vi "ReadIO.vi"(0 "ArrayPairs In":T5={"iStatus"={"Index"=0, "Value"=0.0}, "TIME"={"Index"=1, "Value"=0.0}, "DT"={"Index"=2, "Value"=0.0}, "Blade1PitchPos_rad"={"Index"=3, "Value"=0.0}, "VS_MECHGENPWR"={"Index"=13, "Value"=0.0}, "VS_GENPWR"={"Index"=14, "Value"=0.0}, "GEN_SPEED"={"Index"=19, "Value"=0.0}, "ROTOR_SPEED"={"Index"=20, "Value"=0.0}, "GENTQMEAS"={"Index"=22, "Value"=0.0}, "Y_M"={"Index"=23, "Value"=0.0}, "HORWINDV"={"Index"=26, "Value"=0.0}, "ROOTMOOP1"={"Index"=29, "Value"=0.0}, "ROOTMOOP2"={"Index"=30, "Value"=0.0}, "Blade2PitchPos_rad"={"Index"=32, "Value"=0.0}, "Blade3PitchPos_rad"={"Index"=33, "Value"=0.0}, "ROOTMOOP3"={"Index"=31, "Value"=0.0}, "AVCMSG_SIZE"={"Index"=48, "Value"=0.0}, "INFILE_SIZE "={"Index"=49, "Value"=0.0}, "OUTFILE_SIZE "={"Index"=50, "Value"=0.0}, "FA_ACC"={"Index"=52, "Value"=0.0}, "NUM_BLADES"={"Index"=60, "Value"=0.0}, "BladePitchSetpoint_rad"={"Index"=44, "Value"=0.0}, "TorqueSetpoint_Nm"={"Index"=46, "Value"=0.0}, "OUT_AEROTQ"={"Index"=89, "Value"=0.0}, "Out.RotSpeed "={"Index"=92, "Value"=0.0}, "Out.DEBUG"={"Index"=93, "Value"=0.0}}, 1 "PitchAxis1State":T2, 2 "PitchAxis2State":T2, 3 "PitchAxis3State":T2, 5 "IO Signals In":T3, 9 "ROSCO Params In":T4, 11 "error in":errorcluster, 12 "zeroRotorPos":bool) -> (4 "ArrayPairs Out":T5={"iStatus"={"Index"=0, "Value"=0.0}, "TIME"={"Index"=1, "Value"=0.0}, "DT"={"Index"=2, "Value"=0.0}, "Blade1PitchPos_rad"={"Index"=3, "Value"=0.0}, "VS_MECHGENPWR"={"Index"=13, "Value"=0.0}, "VS_GENPWR"={"Index"=14, "Value"=0.0}, "GEN_SPEED"={"Index"=19, "Value"=0.0}, "ROTOR_SPEED"={"Index"=20, "Value"=0.0}, "GENTQMEAS"={"Index"=22, "Value"=0.0}, "Y_M"={"Index"=23, "Value"=0.0}, "HORWINDV"={"Index"=26, "Value"=0.0}, "ROOTMOOP1"={"Index"=29, "Value"=0.0}, "ROOTMOOP2"={"Index"=30, "Value"=0.0}, "Blade2PitchPos_rad"={"Index"=32, "Value"=0.0}, "Blade3PitchPos_rad"={"Index"=33, "Value"=0.0}, "ROOTMOOP3"={"Index"=31, "Value"=0.0}, "AVCMSG_SIZE"={"Index"=48, "Value"=0.0}, "INFILE_SIZE "={"Index"=49, "Value"=0.0}, "OUTFILE_SIZE "={"Index"=50, "Value"=0.0}, "FA_ACC"={"Index"=52, "Value"=0.0}, "NUM_BLADES"={"Index"=60, "Value"=0.0}, "BladePitchSetpoint_rad"={"Index"=44, "Value"=0.0}, "TorqueSetpoint_Nm"={"Index"=46, "Value"=0.0}, "OUT_AEROTQ"={"Index"=89, "Value"=0.0}, "Out.RotSpeed "={"Index"=92, "Value"=0.0}, "Out.DEBUG"={"Index"=93, "Value"=0.0}}, 6 "IO Signals Out":T3, 10 "ROSCO Params Out":T4, 14 "Torque RAW (V)":dbl, 15 "error out":errorcluster)   [LabVIEW 2018]
uses:
  Clusters/ArrayPairs.ctl
  Clusters/SwapArrayCluster.ctl
  Clusters/RoscoParams.ctl
  Clusters/IOSignals.ctl
  Clusters/ElmoState.ctl
  Clusters/AnemometerData.ctl
  Clusters/SimulationConstants.ctl
panel:
  in  "Anemometer Data":T1
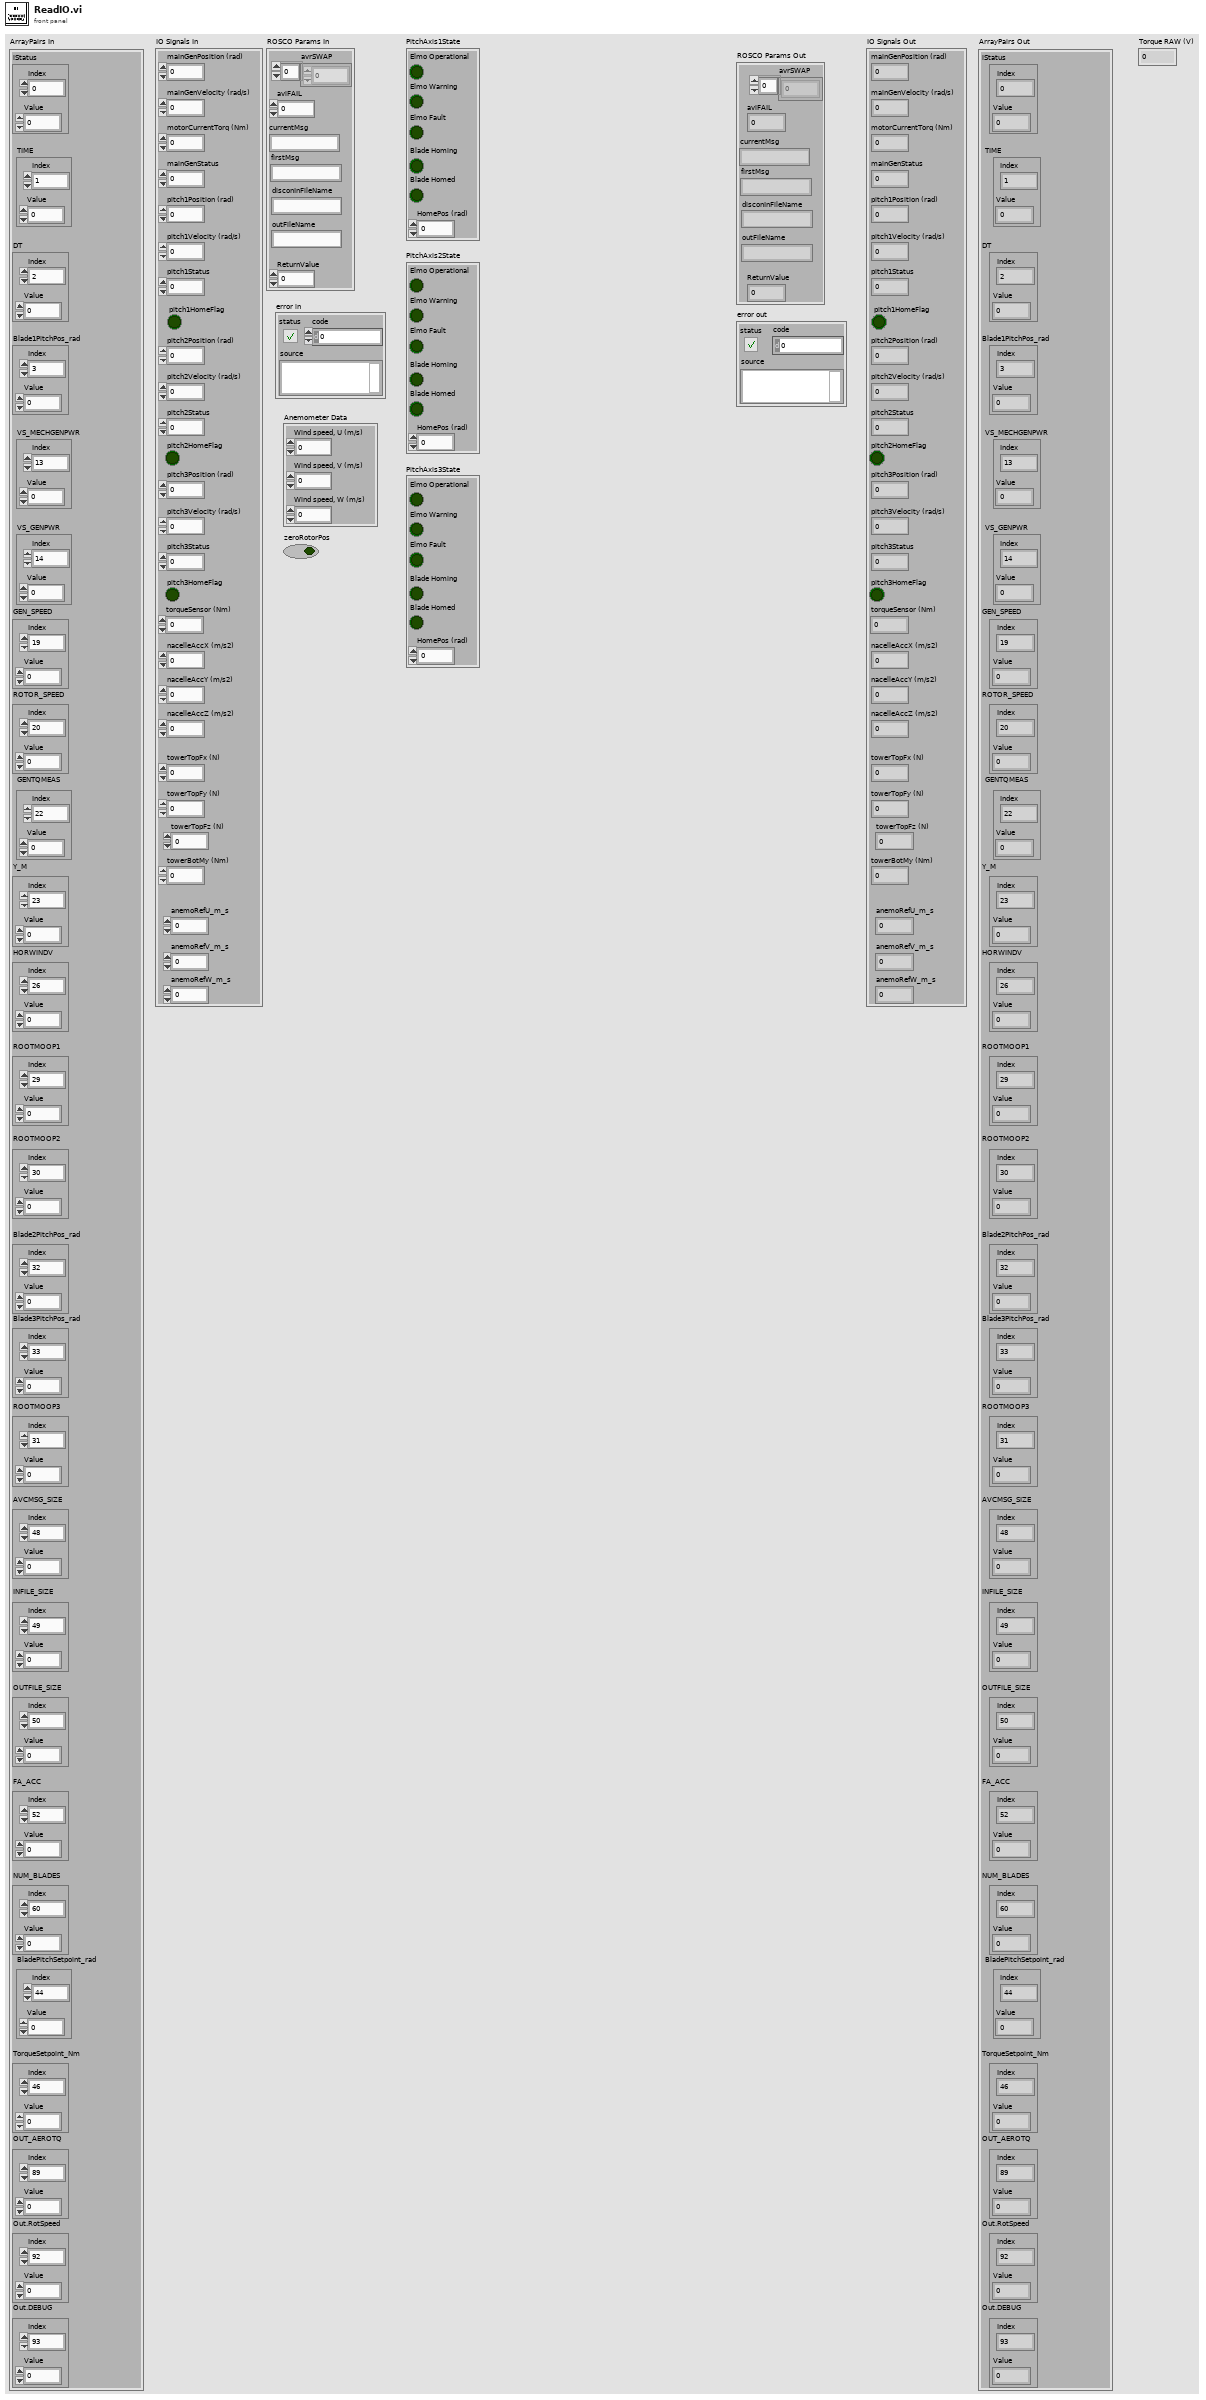
[diagram p1: front panel]
types:
  T1 = typedef "AnemometerData.ctl" = cluster{"Wind speed, U (m/s)":dbl, "Wind speed, V (m/s)":dbl, "Wind speed, W (m/s)":dbl}
  T2 = typedef "ElmoState.ctl" = cluster{"Elmo Operational":bool, "Elmo Warning":bool, "Elmo Fault":bool, "Blade Homed":bool, "Blade Homing":bool, "HomePos (rad)":dbl}
  T3 = typedef "IOSignals.ctl" = cluster{"mainGenPosition (rad)":dbl, "motorCurrentTorq (Nm)":dbl, "mainGenVelocity (rad/s)":dbl, "mainGenStatus":u16, "pitch1Position (rad)":dbl, "pitch1Velocity (rad/s)":dbl, "pitch1Status":u16, "pitch2Position (rad)":dbl, "pitch2Velocity (rad/s)":dbl, "pitch2Status":u16, "pitch3Position (rad)":dbl, "pitch3Velocity (rad/s)":dbl, "pitch3Status":u16, "torqueSensor (Nm)":dbl, "nacelleAccX (m/s2)":dbl, "nacelleAccY (m/s2)":dbl, "nacelleAccZ (m/s2)":dbl, "pitch1HomeFlag":bool, "pitch2HomeFlag":bool, "pitch3HomeFlag":bool, "towerTopFx (N)":dbl, "towerTopFy (N)":dbl, "towerTopFz (N)":dbl, "towerBotMy (Nm)":dbl, "anemoRefU_m_s":dbl, "anemoRefV_m_s":dbl, "anemoRefW_m_s":dbl}
  T4 = typedef "RoscoParams.ctl" = cluster{"avrSWAP":dbl[], "aviFAIL":i32, "currentMsg":string, "ReturnValue":i32, "disconInFileName":string, "outFileName":string, "firstMsg":string}
  T5 = typedef "ArrayPairs.ctl" = cluster{"iStatus":T6, "TIME":T6, "DT":T6, "Blade1PitchPos_rad":T6, "VS_MECHGENPWR":T6, "VS_GENPWR":T6, "GEN_SPEED":T6, "ROTOR_SPEED":T6, "GENTQMEAS":T6, "Y_M":T6, "HORWINDV":T6, "ROOTMOOP1":T6, "ROOTMOOP2":T6, "Blade2PitchPos_rad":T6, "Blade3PitchPos_rad":T6, "ROOTMOOP3":T6, "AVCMSG_SIZE":T6, "INFILE_SIZE ":T6, "OUTFILE_SIZE ":T6, "FA_ACC":T6, "NUM_BLADES":T6, "BladePitchSetpoint_rad":T6, "TorqueSetpoint_Nm":T6, "OUT_AEROTQ":T6, "Out.RotSpeed ":T6, "Out.DEBUG":T6}
  T6 = typedef "SwapArrayCluster.ctl" = cluster{"Index":i32, "Value":dbl}
  T7 = typedef "SimulationConstants.ctl" = cluster{"nGear":dbl, "rotorRadius":sgl, "numBlades":i32, "scaleFactor":dbl, "roscoInitMinSpeed_rad_s":dbl, "roscoInitMinTorqueFS_Nm":dbl, "beckhoff16bit":dbl, "beckhoff24BitExt":i32, "BX824Bit":i32, "rotorTorqueScale_Nm_V":dbl, "rotorTorqueOfst_Nm":dbl, "rangeEL3104V":dbl, "nacelleAccELM3604V":dbl, "nacelleAccScaleX_m_s2_V":dbl, "nacelleAccOfstX_m_s2":dbl, "nacelleAccScaleY_m_s2_V":dbl, "nacelleAccOfstY_m_s2":dbl, "nacelleAccScaleZ_m_s2_V":dbl, "nacelleAccOfstZ_m_s2":dbl, "cyberGearRatio":dbl, "cyberLinesPerRev":dbl, "cyberRatedTorque":dbl, "towerTopForceScale":dbl, "towerTopTorqueScale":dbl, "plcSetpointScaling_norm2VFD":dbl, "towerBotScaleMy_Nm_V":dbl, "towerBotOfstMy_Nm":dbl, "towerTopScaleXaxis_N_V":dbl, "towerTopOfstXaxis_N":dbl, "towerTopScaleYaxis_N_V":dbl, "towerTopOfstYaxis_N":dbl, "pitchFlagOffset_deg":dbl, "anemWindSpeedScaleU_m_s_m_s":dbl, "anemWindSpeedOfstU_m_s":dbl, "anemWindSpeedScaleV_m_s_m_s":dbl, "anemWindSpeedOfstV_m_s":dbl, "anemWindSpeedScaleW_m_s_m_s":dbl, "anemWindSpeedOfstW_m_s":dbl, "anemWindSpeedScaleTSI1_m_s_V":dbl, "anemWindSpeedOfstTSI1_m_s":dbl}
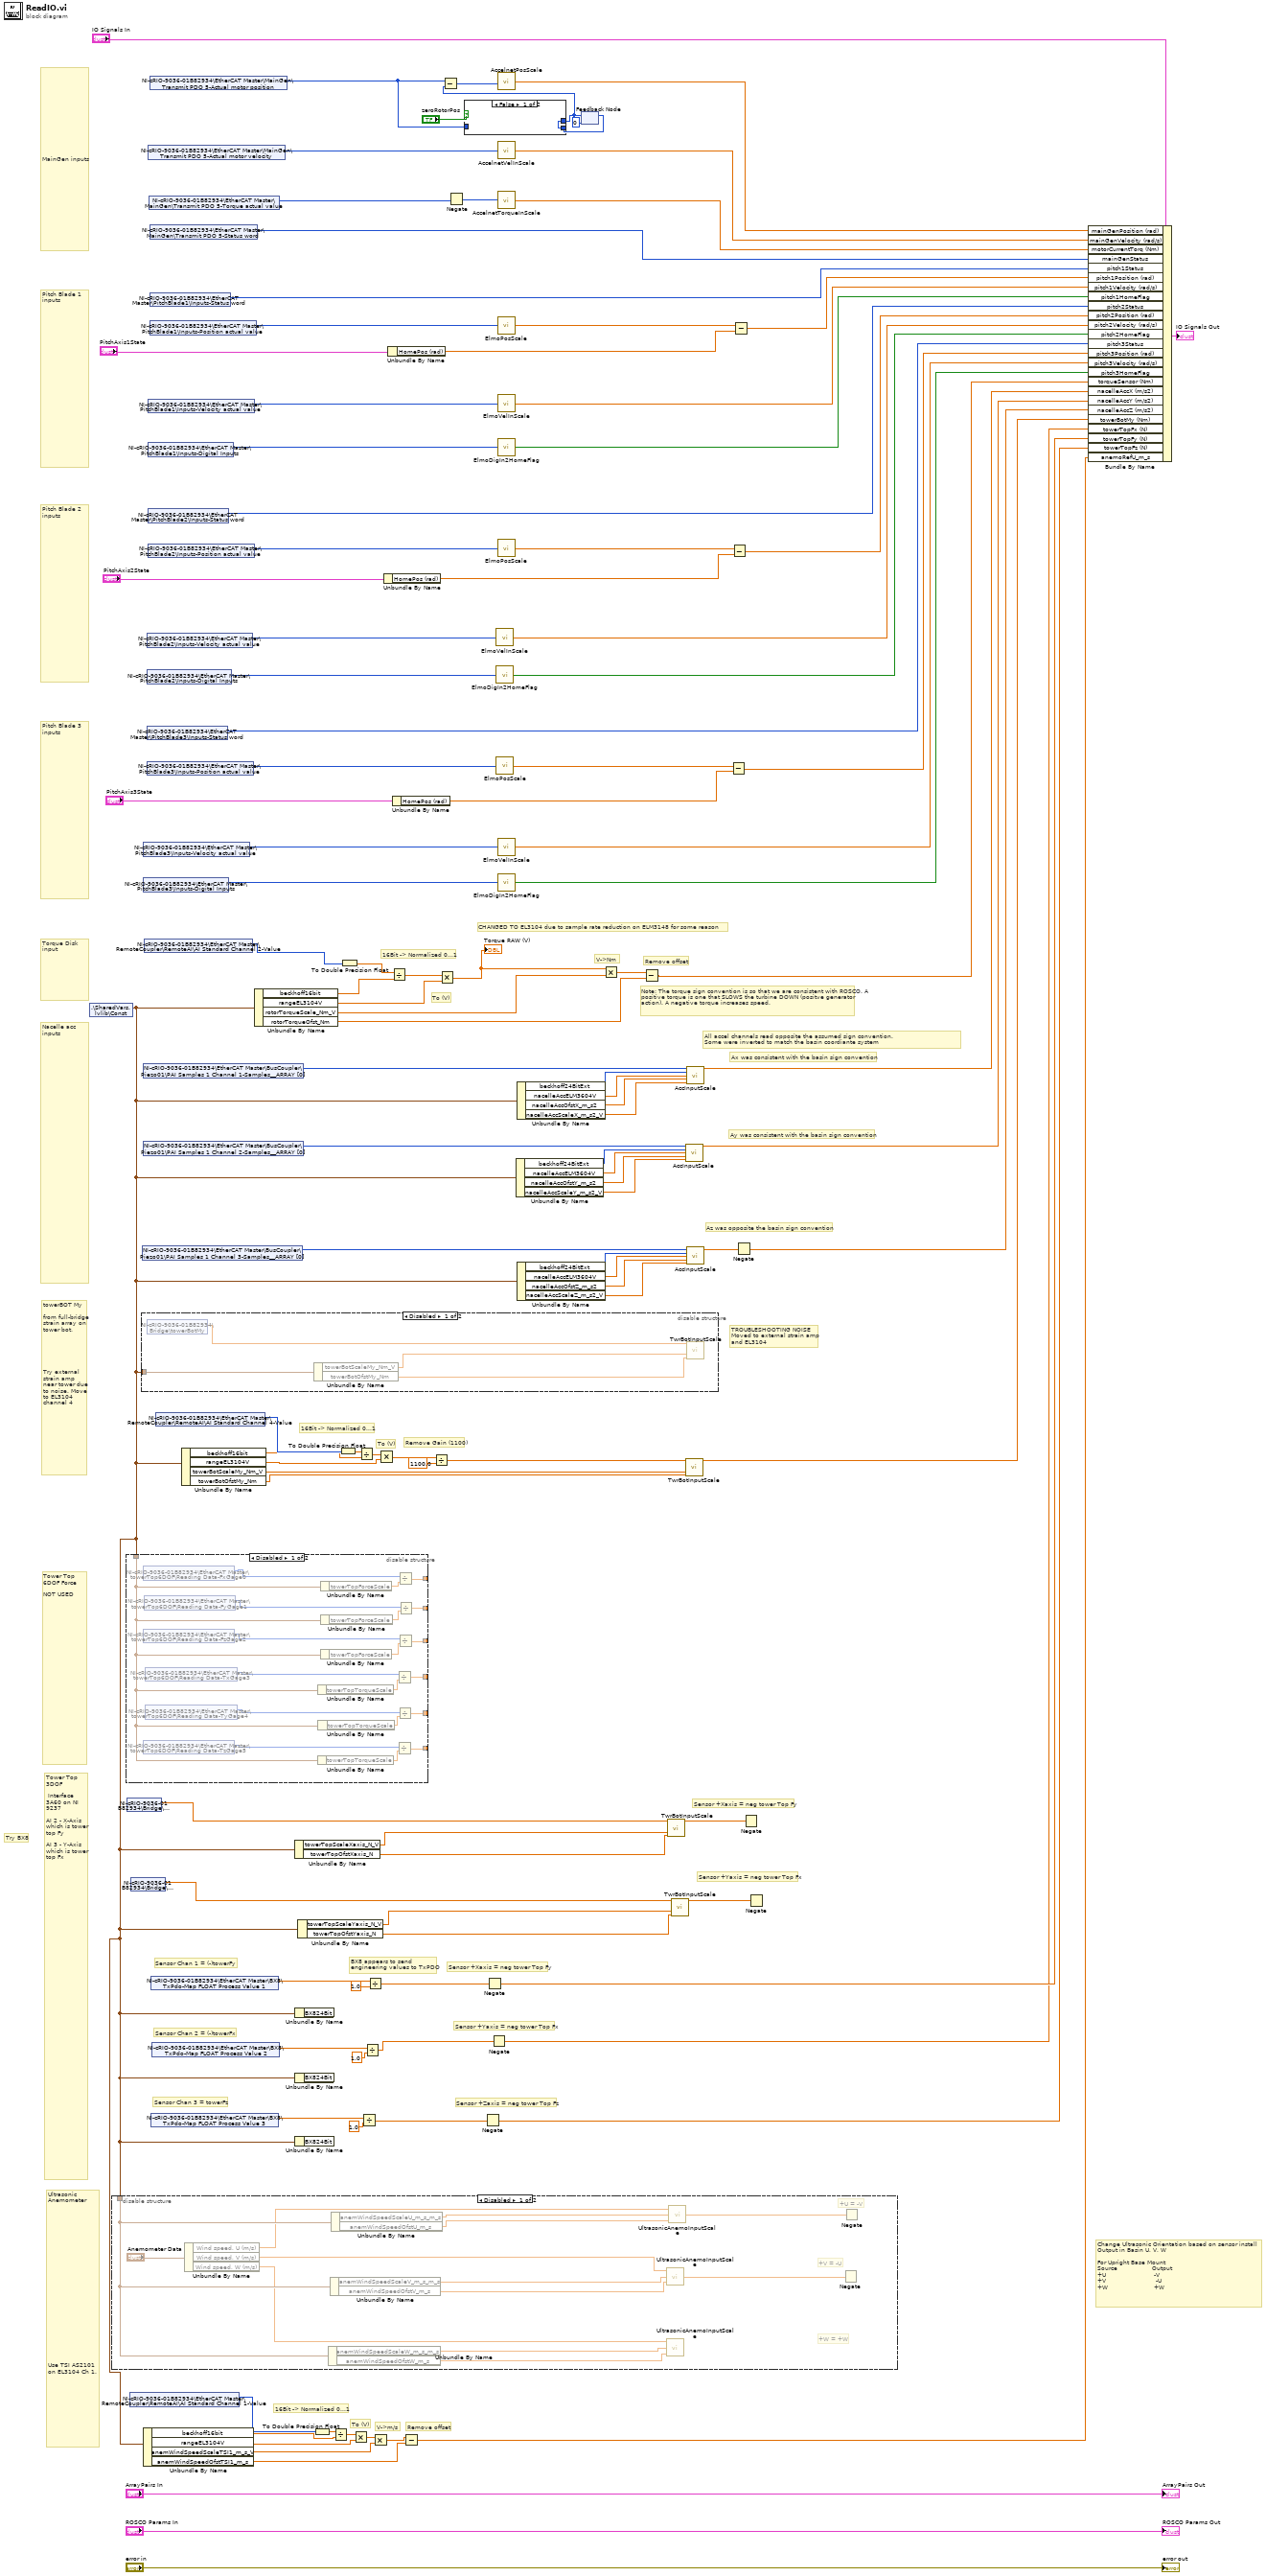
[diagram p0: block diagram]
diagram:
  # "TROUBLESHOOTING NOISE\nMoved to external strain amp\nand EL3104"
  # "Remove Gain (1100)"
  # "To (V)"
  # "16Bit -> Normalized 0...1"
  # "Sensor +Zaxis = neg tower Top Fz"
  # "BX8 appears to send \nengineering values to TxPDO"
  # "Sensor +Yaxis = neg tower Top Fx"
  # "Sensor +Xaxis = neg tower Top Fy"
  # "Sensor Chan 3 = towerFz"
  # "Sensor Chan 2 = (-)towerFx"
  # "Sensor Chan 1 = (-)towerFy"
  # "Try BX8"
  # "Remove offset"
  # "V->m/s"
  # "To (V)"
  # "16Bit -> Normalized 0...1"
  # "Ultrasonic Anemometer\n\n\n\n\n\n\n\n\n\n\n\n\n\n\n\n\n\n\n\n\n\n\n\n\n\n\nUse TSI AS2101\non EL3104 Ch 1."
  # "Remove offset"
  # "CHANGED TO EL3104 due to sample rate reduction on ELM3148 for some reason"
  # "Change Ultrasonic Orientation based on sensor install\nOutput in Basin U, V, W\n\nFor Upright Base Mount\nSource                  Output\n+U                         -V\n+V                          -U\n+W                        +W"
  # "All accel channels read opposite the assumed sign convention. \nSome were inverted to match the basin coordiante system"
  # "Az was opposite the basin sign convention"
  # "Ay was consistent with the basin sign convention"
  # "Ax was consistent with the basin sign convention"
  # "Sensor +Yaxis = neg tower Top Fx"
  # "Sensor +Xaxis = neg tower Top Fy"
  # "Tower Top\n3DOF\n\n Interface 3A60 on NI 9237\n\nAI 2 - X-Axis which is tower top Fy\n\nAI 3 - Y-Axis which is tower top Fx"
  # "towerBOT My\n\nfrom full-bridge strain array on tower bot.\n\n\n\n\n\n\nTry external strain amp near tower due to noise. Move to EL3104 channel 4"
  # "Tower Top\n6DOF Force\n\nNOT USED"
  # "Nacelle acc inputs"
  # "Torque Disk input"
  # "Pitch Blade 3 inputs"
  # "Pitch Blade 2 inputs"
  # "Pitch Blade 1 inputs"
  # "MainGen inputs"
  # "V->Nm"
  # "To (V)"
  # "16Bit -> Normalized 0...1"
  # "Note: The torque sign convention is so that we are consistent with ROSCO. A positive torque is one that SLOWS the turbine DOWN (positve generator action). A negative torque increases speed."
  n1 = shared-variable ".\\SharedVars.lvlib\\Const"() -> (w13:T7)  [unwired: 1 in, 1 out]
  n2 = disable-structure shown="Disabled" {
    disable-tunnel: w13 -> [w132 _]
    frame Disabled {
      # "+V = -U"
      # "+W = +W"
      # "+U = -V"
      n3 = Unbundle By Name("Anemometer Data") -> ("Wind speed, U (m/s)"=w122:dbl, "Wind speed, V (m/s)"=w121:dbl, "Wind speed, W (m/s)"=w120:dbl)
      n4 = Unbundle By Name(w132) -> ("anemWindSpeedScaleW_m_s_m_s"=w127:dbl, "anemWindSpeedOfstW_m_s"=w126:dbl)
      n5 = Unbundle By Name(w132) -> ("anemWindSpeedScaleV_m_s_m_s"=w129:dbl, "anemWindSpeedOfstV_m_s"=w128:dbl)
      n6 = Unbundle By Name(w132) -> ("anemWindSpeedScaleU_m_s_m_s"=w131:dbl, "anemWindSpeedOfstU_m_s"=w130:dbl)
      n7 = call "UltrasonicAnemoInputScale.vi"("Wind Speed Ofst (m/s)"=w128, "Wind Speed Scale (m/s per m/s)"=w129, "Raw Wind Speed (m/s)"=w121) -> ("Wind Speed (m/s)"=w124:dbl)
      n8 = call "UltrasonicAnemoInputScale.vi"("Wind Speed Ofst (m/s)"=w126, "Wind Speed Scale (m/s per m/s)"=w127, "Raw Wind Speed (m/s)"=w120) -> ()  [unwired: 1 out]
      n9 = call "UltrasonicAnemoInputScale.vi"("Wind Speed Ofst (m/s)"=w130, "Wind Speed Scale (m/s per m/s)"=w131, "Raw Wind Speed (m/s)"=w122) -> ("Wind Speed (m/s)"=w125:dbl)
      n10 = Negate(x=w124) -> ()  [unwired: 1 out]
      n11 = Negate(x=w125) -> ()  [unwired: 1 out]
    }
    frame Enabled {
    }
  }
  n12 = disable-structure shown="Disabled" {
    disable-tunnel: [w139 _] -> _
    disable-tunnel: [w138 _] -> _
    disable-tunnel: [w137 _] -> _
    disable-tunnel: [w136 _] -> _
    disable-tunnel: [w135 _] -> _
    disable-tunnel: [w134 _] -> _
    disable-tunnel: w13 -> [w133 _]
    frame Disabled {
      n13 = shared-variable "NI-cRIO-9036-01B82934\\EtherCAT Master\\towerTop6DOF\\Reading Data-FxGage0"() -> (w145:i32)  [unwired: 1 in, 1 out]
      n14 = shared-variable "NI-cRIO-9036-01B82934\\EtherCAT Master\\towerTop6DOF\\Reading Data-FzGage2"() -> (w143:i32)  [unwired: 1 in, 1 out]
      n15 = shared-variable "NI-cRIO-9036-01B82934\\EtherCAT Master\\towerTop6DOF\\Reading Data-TzGage5"() -> (w140:i32)  [unwired: 1 in, 1 out]
      n16 = shared-variable "NI-cRIO-9036-01B82934\\EtherCAT Master\\towerTop6DOF\\Reading Data-FyGage1"() -> (w144:i32)  [unwired: 1 in, 1 out]
      n17 = shared-variable "NI-cRIO-9036-01B82934\\EtherCAT Master\\towerTop6DOF\\Reading Data-TyGage4"() -> (w141:i32)  [unwired: 1 in, 1 out]
      n18 = shared-variable "NI-cRIO-9036-01B82934\\EtherCAT Master\\towerTop6DOF\\Reading Data-TxGage3"() -> (w142:i32)  [unwired: 1 in, 1 out]
      n19 = Unbundle By Name(w133) -> ("towerTopTorqueScale"=w148:dbl)
      n20 = Unbundle By Name(w133) -> ("towerTopTorqueScale"=w146:dbl)
      n21 = Unbundle By Name(w133) -> ("towerTopTorqueScale"=w147:dbl)
      n22 = Unbundle By Name(w133) -> ("towerTopForceScale"=w151:dbl)
      n23 = Unbundle By Name(w133) -> ("towerTopForceScale"=w149:dbl)
      n24 = Unbundle By Name(w133) -> ("towerTopForceScale"=w150:dbl)
      n25 = Divide(x=w142, y=w148) -> (x/y=w137:dbl)
      n26 = Divide(x=w140, y=w146) -> (x/y=w139:dbl)
      n27 = Divide(x=w141, y=w147) -> (x/y=w138:dbl)
      n28 = Divide(x=w145, y=w151) -> (x/y=w134:dbl)
      n29 = Divide(x=w143, y=w149) -> (x/y=w136:dbl)
      n30 = Divide(x=w144, y=w150) -> (x/y=w135:dbl)
    }
    frame Enabled {
    }
  }
  n31 = shared-variable "NI-cRIO-9036-01B82934\\Bridge\\AI2"() -> (w58:dbl)  [unwired: 1 in, 1 out]
  n32 = shared-variable "NI-cRIO-9036-01B82934\\EtherCAT Master\\RemoteCoupler\\RemoteAI\\AI Standard Channel 1-Value"() -> (w36:i16)  [unwired: 1 in, 1 out]
  n33 = shared-variable "NI-cRIO-9036-01B82934\\Bridge\\AI3"() -> (w55:dbl)  [unwired: 1 in, 1 out]
  n34 = disable-structure shown="Disabled" {
    disable-tunnel: w13 -> [w152 _]
    frame Disabled {
      n35 = shared-variable "NI-cRIO-9036-01B82934\\Bridge\\towerBotMy"() -> (w155:dbl)  [unwired: 1 in, 1 out]
      n36 = Unbundle By Name(w152) -> ("towerBotScaleMy_Nm_V"=w154:dbl, "towerBotOfstMy_Nm"=w153:dbl)
      n37 = call "TwrBotInputScale.vi"("Signal (V)"=w155, "Scale (Nm/V)"=w154, "Offset (Nm)"=w153) -> ()  [unwired: 12 in, 1 out]
    }
    frame Enabled {
    }
  }
  n38 = shared-variable "NI-cRIO-9036-01B82934\\EtherCAT Master\\BusCoupler\\Piezo01\\PAI Samples 1 Channel 3-Samples__ARRAY [0]"() -> (w76:i32)  [unwired: 1 in, 1 out]
  n39 = Unbundle By Name(w13) -> ("beckhoff16bit"=w35:dbl, "rangeEL3104V"=w34:dbl, "anemWindSpeedScaleTSI1_m_s_V"=w33:dbl, "anemWindSpeedOfstTSI1_m_s"=w32:dbl)
  n40 = shared-variable "NI-cRIO-9036-01B82934\\EtherCAT Master\\PitchBlade3\\Inputs-Velocity actual value"() -> (w105:i32)  [unwired: 1 in, 1 out]
  n41 = shared-variable "NI-cRIO-9036-01B82934\\EtherCAT Master\\PitchBlade3\\Inputs-Digital Inputs"() -> (w64:i32)  [unwired: 1 in, 1 out]
  n42 = shared-variable "NI-cRIO-9036-01B82934\\EtherCAT Master\\BusCoupler\\Piezo01\\PAI Samples 1 Channel 1-Samples__ARRAY [0]"() -> (w90:i32)  [unwired: 1 in, 1 out]
  n43 = shared-variable "NI-cRIO-9036-01B82934\\EtherCAT Master\\BusCoupler\\Piezo01\\PAI Samples 1 Channel 2-Samples__ARRAY [0]"() -> (w77:i32)  [unwired: 1 in, 1 out]
  n44 = shared-variable "NI-cRIO-9036-01B82934\\EtherCAT Master\\RemoteCoupler\\RemoteAI\\AI Standard Channel 2-Value"() -> (w47:i16)  [unwired: 1 in, 1 out]
  n45 = shared-variable "NI-cRIO-9036-01B82934\\EtherCAT Master\\PitchBlade2\\Inputs-Velocity actual value"() -> (w108:i32)  [unwired: 1 in, 1 out]
  n46 = shared-variable "NI-cRIO-9036-01B82934\\EtherCAT Master\\PitchBlade2\\Inputs-Digital Inputs"() -> (w65:i32)  [unwired: 1 in, 1 out]
  n47 = shared-variable "NI-cRIO-9036-01B82934\\EtherCAT Master\\PitchBlade3\\Inputs-Status word"() -> (w96:u16)  [unwired: 1 in, 1 out]
  n48 = shared-variable "NI-cRIO-9036-01B82934\\EtherCAT Master\\PitchBlade3\\Inputs-Position actual value"() -> (w106:i32)  [unwired: 1 in, 1 out]
  n49 = shared-variable "NI-cRIO-9036-01B82934\\EtherCAT Master\\PitchBlade1\\Inputs-Velocity actual value"() -> (w112:i32)  [unwired: 1 in, 1 out]
  n50 = shared-variable "NI-cRIO-9036-01B82934\\EtherCAT Master\\PitchBlade1\\Inputs-Digital Inputs"() -> (w75:i32)  [unwired: 1 in, 1 out]
  n51 = shared-variable "NI-cRIO-9036-01B82934\\EtherCAT Master\\PitchBlade2\\Inputs-Status word"() -> (w101:u16)  [unwired: 1 in, 1 out]
  n52 = shared-variable "NI-cRIO-9036-01B82934\\EtherCAT Master\\PitchBlade2\\Inputs-Position actual value"() -> (w107:i32)  [unwired: 1 in, 1 out]
  n53 = shared-variable "NI-cRIO-9036-01B82934\\EtherCAT Master\\MainGen\\Transmit PDO 5-Actual motor velocity"() -> (w63:i32)  [unwired: 1 in, 1 out]
  n54 = shared-variable "NI-cRIO-9036-01B82934\\EtherCAT Master\\MainGen\\Transmit PDO 5-Torque actual value"() -> (w109:i16)  [unwired: 1 in, 1 out]
  n55 = shared-variable "NI-cRIO-9036-01B82934\\EtherCAT Master\\MainGen\\Transmit PDO 5-Actual motor position"() -> (w5:i32)  [unwired: 1 in, 1 out]
  n56 = shared-variable "NI-cRIO-9036-01B82934\\EtherCAT Master\\MainGen\\Transmit PDO 5-Status word"() -> (w115:u16)  [unwired: 1 in, 1 out]
  n57 = shared-variable "NI-cRIO-9036-01B82934\\EtherCAT Master\\PitchBlade1\\Inputs-Status word"() -> (w103:u16)  [unwired: 1 in, 1 out]
  n58 = shared-variable "NI-cRIO-9036-01B82934\\EtherCAT Master\\PitchBlade1\\Inputs-Position actual value"() -> (w113:i32)  [unwired: 1 in, 1 out]
  n59 = shared-variable "NI-cRIO-9036-01B82934\\EtherCAT Master\\BX8\\TxPdo-Map FLOAT Process Value 1"() -> (w30:sgl)  [unwired: 1 in, 1 out]
  n60 = shared-variable "NI-cRIO-9036-01B82934\\EtherCAT Master\\BX8\\TxPdo-Map FLOAT Process Value 3"() -> (w28:sgl)  [unwired: 1 in, 1 out]
  n61 = shared-variable "NI-cRIO-9036-01B82934\\EtherCAT Master\\BX8\\TxPdo-Map FLOAT Process Value 2"() -> (w29:sgl)  [unwired: 1 in, 1 out]
  n62 = shared-variable "NI-cRIO-9036-01B82934\\EtherCAT Master\\RemoteCoupler\\RemoteAI\\AI Standard Channel 4-Value"() -> (w16:i16)  [unwired: 1 in, 1 out]
  n63 = Unbundle By Name(w13) -> ("beckhoff16bit"=w15:dbl, "rangeEL3104V"=w14:dbl, "towerBotScaleMy_Nm_V"=w9:dbl, "towerBotOfstMy_Nm"=w8:dbl)
  n64 = Unbundle By Name(w13) -> ("beckhoff16bit"=w46:dbl, "rangeEL3104V"=w91:dbl, "rotorTorqueScale_Nm_V"=w44:dbl, "rotorTorqueOfst_Nm"=w42:dbl)
  n65 = Unbundle By Name(w13) -> ("towerTopScaleXaxis_N_V"=w60:dbl, "towerTopOfstXaxis_N"=w59:dbl)
  n66 = Unbundle By Name(w13) -> ()  [unwired: 1 out]
  n67 = Unbundle By Name(w13) -> ()  [unwired: 1 out]
  n68 = Unbundle By Name(w13) -> ()  [unwired: 1 out]
  n69 = Unbundle By Name(w13) -> ("towerTopScaleYaxis_N_V"=w57:dbl, "towerTopOfstYaxis_N"=w56:dbl)
  n70 = To Double Precision Float(number=w36) -> (double precision float=w39:dbl)
  n71 = Divide(x=w39, y=w35) -> (x/y=w40:dbl)
  n72 = To Double Precision Float(number=w16) -> (double precision float=w17:dbl)
  n73 = To Double Precision Float(number=w47) -> (double precision float=w48:dbl)
  n74 = Multiply(x=w40, y=w34) -> (x*y=w38:dbl)
  n75 = Divide(x=w17, y=w15) -> (x/y=w18:dbl)
  n76 = Divide(x=w28, y=sgl 1.0) -> (x/y=w20:sgl)
  n77 = Divide(x=w29, y=sgl 1.0) -> (x/y=w25:sgl)
  n78 = Divide(x=w30, y=sgl 1.0) -> (x/y=w27:sgl)
  n79 = Multiply(x=w38, y=w33) -> (x*y=w37:dbl)
  n80 = Multiply(x=w18, y=w14) -> (x*y=w11:dbl)
  n81 = Unbundle By Name("PitchAxis2State") -> ("HomePos (rad)"=w68:dbl)
  n82 = Unbundle By Name("PitchAxis1State") -> ("HomePos (rad)"=w70:dbl)
  n83 = Divide(x=w48, y=w46) -> (x/y=w92:dbl)
  n84 = Unbundle By Name("PitchAxis3State") -> ("HomePos (rad)"=w66:dbl)
  n85 = Subtract(x=w37, y=w32) -> (x-y=w31:dbl)
  n86 = Divide(x=w11, y=1100.0) -> (x/y=w10:dbl)
  n87 = Multiply(x=w92, y=w91) -> (x*y=w45:dbl)
  "Torque RAW (V)" <- w45
  n88 = Negate(x=w109) -> (-x=w62:i16)
  n89 = Negate(x=w20) -> (-x=w19:sgl)
  n90 = Negate(x=w27) -> (-x=w26:sgl)
  n91 = Negate(x=w25) -> (-x=w24:sgl)
  n92 = call "ElmoVelInScale.vi"("Elmo eCAT vel (ticks/s)"=w108) -> ("Elmo vel (rad/s)"=w97:dbl)
  n93 = call "ElmoDigIn2HomeFlag.vi"("Digital Input (I32)"=w65) -> ("Home Flag"=w73:bool)
  n94 = call "ElmoPosScale.vi"("Elmo eCAT pos (ticks)"=w106) -> ("Elmo pos (rad)"=w95:dbl)
  n95 = call "AccelnetVelInScale.vi"("Acelnet eCAT vel"=w63) -> ("Shaft vel (rad/s)"=w110:dbl)
  n96 = call "AccelnetTorqueInScale.vi"("Torque (Raw from drive)"=w62) -> ("Torque (Nm)"=w61:dbl)
  n97 = call "ElmoPosScale.vi"("Elmo eCAT pos (ticks)"=w113) -> ("Elmo pos (rad)"=w111:dbl)
  n98 = call "ElmoVelInScale.vi"("Elmo eCAT vel (ticks/s)"=w112) -> ("Elmo vel (rad/s)"=w98:dbl)
  n99 = call "ElmoDigIn2HomeFlag.vi"("Digital Input (I32)"=w75) -> ("Home Flag"=w74:bool)
  n100 = call "ElmoPosScale.vi"("Elmo eCAT pos (ticks)"=w107) -> ("Elmo pos (rad)"=w99:dbl)
  n101 = call "ElmoVelInScale.vi"("Elmo eCAT vel (ticks/s)"=w105) -> ("Elmo vel (rad/s)"=w93:dbl)
  n102 = call "ElmoDigIn2HomeFlag.vi"("Digital Input (I32)"=w64) -> ("Home Flag"=w72:bool)
  n103 = Unbundle By Name(w13) -> ("beckhoff24BitExt"=w82:i32, "nacelleAccELM3604V"=w83:dbl, "nacelleAccOfstY_m_s2"=w84:dbl, "nacelleAccScaleY_m_s2_V"=w85:dbl)
  n104 = Unbundle By Name(w13) -> ("beckhoff24BitExt"=w89:i32, "nacelleAccELM3604V"=w88:dbl, "nacelleAccOfstX_m_s2"=w87:dbl, "nacelleAccScaleX_m_s2_V"=w86:dbl)
  n105 = Unbundle By Name(w13) -> ("beckhoff24BitExt"=w81:i32, "nacelleAccELM3604V"=w80:dbl, "nacelleAccOfstZ_m_s2"=w79:dbl, "nacelleAccScaleZ_m_s2_V"=w78:dbl)
  n106 = feedback #1(0) -> (w3:i32)
  n107 = case shown="False" "zeroRotorPos" {
    tunnel: w5 -> [_ w157]
    tunnel: [w156 w157] -> w1
    tunnel: w3 -> [w156 _]
    frame False {
    }
    frame True {
    }
  }
  n108 = Subtract(x=w5, y=w1) -> (x-y=w6:i32)
  n109 = call "AccelnetPosScale.vi"("Accelnet eCAT Pos"=w6) -> ("Shaft Pos (rad)"=w114:dbl)
  n110 = feedback-in #1(w1) -> ()
  n111 = Multiply(x=w45, y=w44) -> (x*y=w43:dbl)
  n112 = Subtract(x=w43, y=w42) -> (x-y=w41:dbl)
  n113 = call "TwrBotInputScale.vi"("Signal (V)"=w58, "Scale (Nm/V)"=w60, "Offset (Nm)"=w59) -> ("Output (Nm)"=w54:dbl)  [unwired: 12 in]
  n114 = call "TwrBotInputScale.vi"("Signal (V)"=w55, "Scale (Nm/V)"=w57, "Offset (Nm)"=w56) -> ("Output (Nm)"=w53:dbl)  [unwired: 12 in]
  n115 = call "AccInputScale.vi"("EtherCATSignal"=w77, "ELM3604MaxBits"=w82, "ELM3604MaxVolts"=w83, "Acc Offset ((m/s2))"=w84, "AccScale ((m/s2)/V)"=w85) -> ("Acc (m/s2)"=w51:dbl)  [unwired: 10 in]
  n116 = call "TwrBotInputScale.vi"("Signal (V)"=w10, "Scale (Nm/V)"=w9, "Offset (Nm)"=w8) -> ("Output (Nm)"=w7:dbl)  [unwired: 12 in]
  n117 = call "AccInputScale.vi"("EtherCATSignal"=w90, "ELM3604MaxBits"=w89, "ELM3604MaxVolts"=w88, "Acc Offset ((m/s2))"=w87, "AccScale ((m/s2)/V)"=w86) -> ("Acc (m/s2)"=w52:dbl)  [unwired: 10 in]
  n118 = call "AccInputScale.vi"("EtherCATSignal"=w76, "ELM3604MaxBits"=w81, "ELM3604MaxVolts"=w80, "Acc Offset ((m/s2))"=w79, "AccScale ((m/s2)/V)"=w78) -> ("Acc (m/s2)"=w50:dbl)  [unwired: 10 in]
  n119 = Subtract(x=w95, y=w66) -> (x-y=w94:dbl)
  n120 = Subtract(x=w99, y=w68) -> (x-y=w100:dbl)
  n121 = Subtract(x=w111, y=w70) -> (x-y=w102:dbl)
  n122 = Negate(x=w50) -> (-x=w49:dbl)
  n123 = Negate(x=w54) -> ()  [unwired: 1 out]
  n124 = Negate(x=w53) -> ()  [unwired: 1 out]
  n125 = Bundle By Name(cluster="IO Signals In", "mainGenPosition (rad)"=w114, "mainGenVelocity (rad/s)"=w110, "motorCurrentTorq (Nm)"=w61, "mainGenStatus"=w115, "pitch1Status"=w103, "pitch1Position (rad)"=w102, "pitch1Velocity (rad/s)"=w98, "pitch1HomeFlag"=w74, "pitch2Status"=w101, "pitch2Position (rad)"=w100, "pitch2Velocity (rad/s)"=w97, "pitch2HomeFlag"=w73, "pitch3Status"=w96, "pitch3Position (rad)"=w94, "pitch3Velocity (rad/s)"=w93, "pitch3HomeFlag"=w72, "torqueSensor (Nm)"=w41, "nacelleAccX (m/s2)"=w52, "nacelleAccY (m/s2)"=w51, "nacelleAccZ (m/s2)"=w49, "towerBotMy (Nm)"=w7, "towerTopFx (N)"=w24, "towerTopFy (N)"=w26, "towerTopFz (N)"=w19, "anemoRefU_m_s"=w31) -> (→"IO Signals Out":T3)
  "error out" <- "error in"
  "ArrayPairs Out" <- "ArrayPairs In"
  "ROSCO Params Out" <- "ROSCO Params In"
